vi "LastDataToFolders.vi"(10 "Inst:Test Name":string, 11 "Last Path":path) -> (2 "Path To TRF Folder":path, 3 "Path to csv Folder":path, 5 "Path to test Folder":path)   [LabVIEW 2022 SP3]
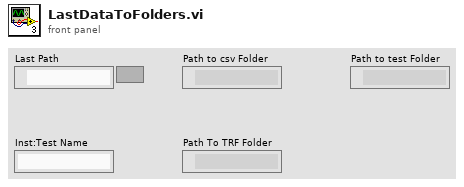
[diagram p1: front panel]
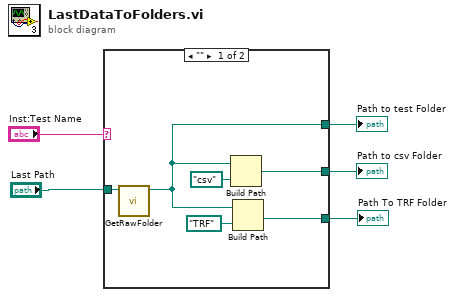
[diagram p0: block diagram]
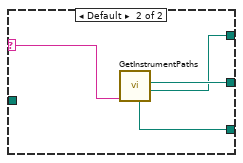
[diagram p2: hidden frame]
diagram:
  n1 = case shown="\"\"" "Inst:Test Name" {
    selector: "Inst:Test Name" -> [_ w14]
    tunnel: [w10 w15] -> w3
    tunnel: [w8 w13] -> w5
    tunnel: [w6 w12] -> w2
    tunnel: "Last Path" -> [w7 _]
    frame "" {
      n2 = call "GetRawFolder.vi"("File name"=w7) -> ("Path to Raw data"=w6:path)  [unwired: 10 in]
      n3 = Build Path(base path=w6, name or relative path=path "csv" ("Path to csv Folder")) -> (appended path=w10:path)
      n4 = Build Path(base path=w6, name or relative path=path "TRF" ("Path to csv Folder")) -> (appended path=w8:path)
    }
    frame Default {
      n5 = call "GetInstrumentPaths.vi"("Instrument"=w14) -> ("Path To Test Folder"=w12:path, "Path to csv Folder"=w15:path, "Path To TRF Folder"=w13:path)  [unwired: 6 in, 2 out]
    }
  }
  "Path To TRF Folder" <- w5
  "Path to csv Folder" <- w3
  "Path to test Folder" <- w2
